vi "PCO_LensControlParameters.vi"() -> (0 "PCO_LensControlParameters":T2 {"dwStatusFlags" format="%x"}, 1 "PCO_LensControlParameters_Raw":T1, 2 "Length":u16, 3 "Raw_Length":u16)   [LabVIEW 2020, in "SDK.lvlib" / "Structures.lvlib"]
doc: "Use this template to build a VI to use as a subVI."
uses:
  Structures.lvlib
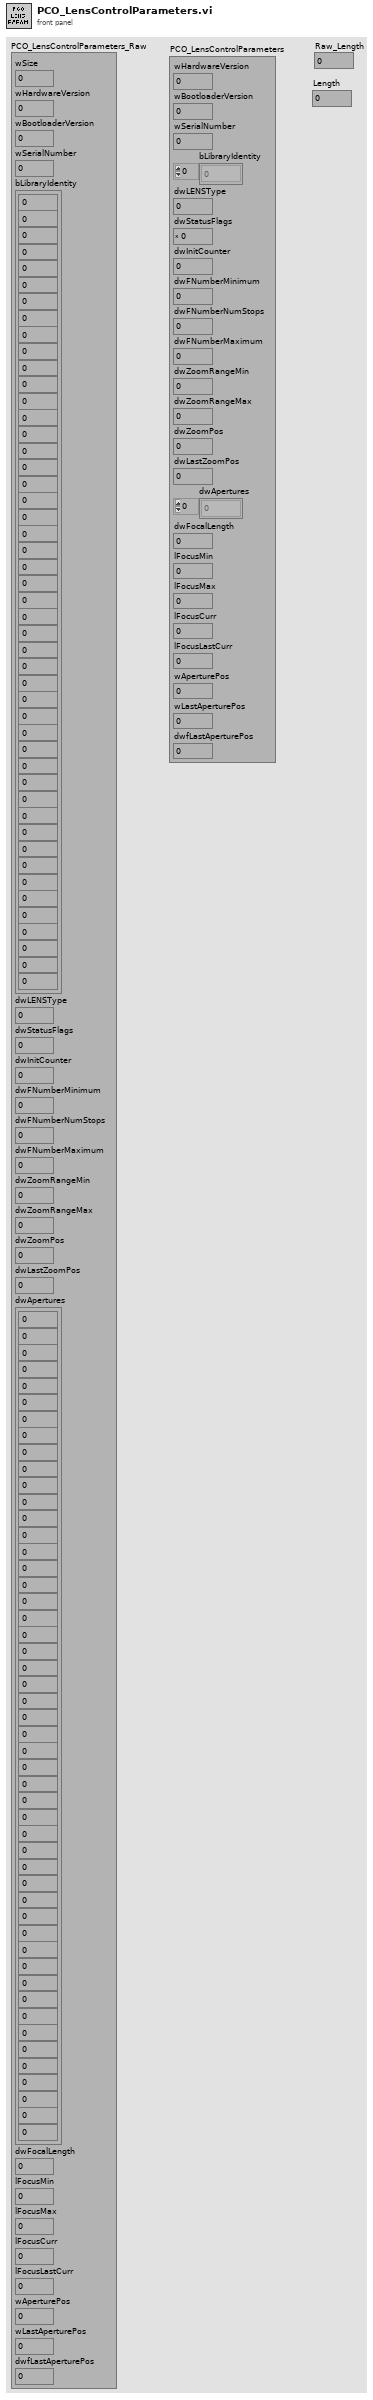
[diagram p1: front panel]
types:
  T1 = cluster{"wSize":u16, "wHardwareVersion":u16, "wBootloaderVersion":u16, "wSerialNumber":u16, "bLibraryIdentity":cluster{u8, u8, u8, u8, u8, u8, u8, u8, u8, u8, u8, u8, u8, u8, u8, u8, u8, u8, u8, u8, u8, u8, u8, u8, u8, u8, u8, u8, u8, u8, u8, u8, u8, u8, u8, u8, u8, u8, u8, u8, u8, u8, u8, u8, u8, u8, u8, u8}, "dwLENSType":u32, "dwStatusFlags":u32, "dwInitCounter":u32, "dwFNumberMinimum":u32, "dwFNumberNumStops":u32, "dwFNumberMaximum":u32, "dwZoomRangeMin":u32, "dwZoomRangeMax":u32, "dwZoomPos":u32, "dwLastZoomPos":u32, "dwApertures":cluster{u32, u32, u32, u32, u32, u32, u32, u32, u32, u32, u32, u32, u32, u32, u32, u32, u32, u32, u32, u32, u32, u32, u32, u32, u32, u32, u32, u32, u32, u32, u32, u32, u32, u32, u32, u32, u32, u32, u32, u32, u32, u32, u32, u32, u32, u32, u32, u32, u32, u32}, "dwFocalLength":u32, "lFocusMin":i32, "lFocusMax":i32, "lFocusCurr":i32, "lFocusLastCurr":i32, "wAperturePos":u16, "wLastAperturePos":u16, "dwfLastAperturePos":u32}
  T2 = cluster{"wHardwareVersion":u16, "wBootloaderVersion":u16, "wSerialNumber":u16, "bLibraryIdentity":u8[], "dwLENSType":u32, "dwStatusFlags":u32, "dwInitCounter":u32, "dwFNumberMinimum":u32, "dwFNumberNumStops":u32, "dwFNumberMaximum":u32, "dwZoomRangeMin":u32, "dwZoomRangeMax":u32, "dwZoomPos":u32, "dwLastZoomPos":u32, "dwApertures":u32[], "dwFocalLength":u32, "lFocusMin":i32, "lFocusMax":i32, "lFocusCurr":i32, "lFocusLastCurr":i32, "wAperturePos":u16, "wLastAperturePos":u16, "dwfLastAperturePos":u32}
  T3 = cluster{u32, u32, u32, u32, u32, u32, u32, u32, u32, u32, u32, u32, u32, u32, u32, u32, u32, u32, u32, u32, u32, u32, u32, u32, u32, u32, u32, u32, u32, u32, u32, u32, u32, u32, u32, u32, u32, u32, u32, u32, u32, u32, u32, u32, u32, u32, u32, u32, u32, u32}
  T4 = cluster{u8, u8, u8, u8, u8, u8, u8, u8, u8, u8, u8, u8, u8, u8, u8, u8, u8, u8, u8, u8, u8, u8, u8, u8, u8, u8, u8, u8, u8, u8, u8, u8, u8, u8, u8, u8, u8, u8, u8, u8, u8, u8, u8, u8, u8, u8, u8, u8}
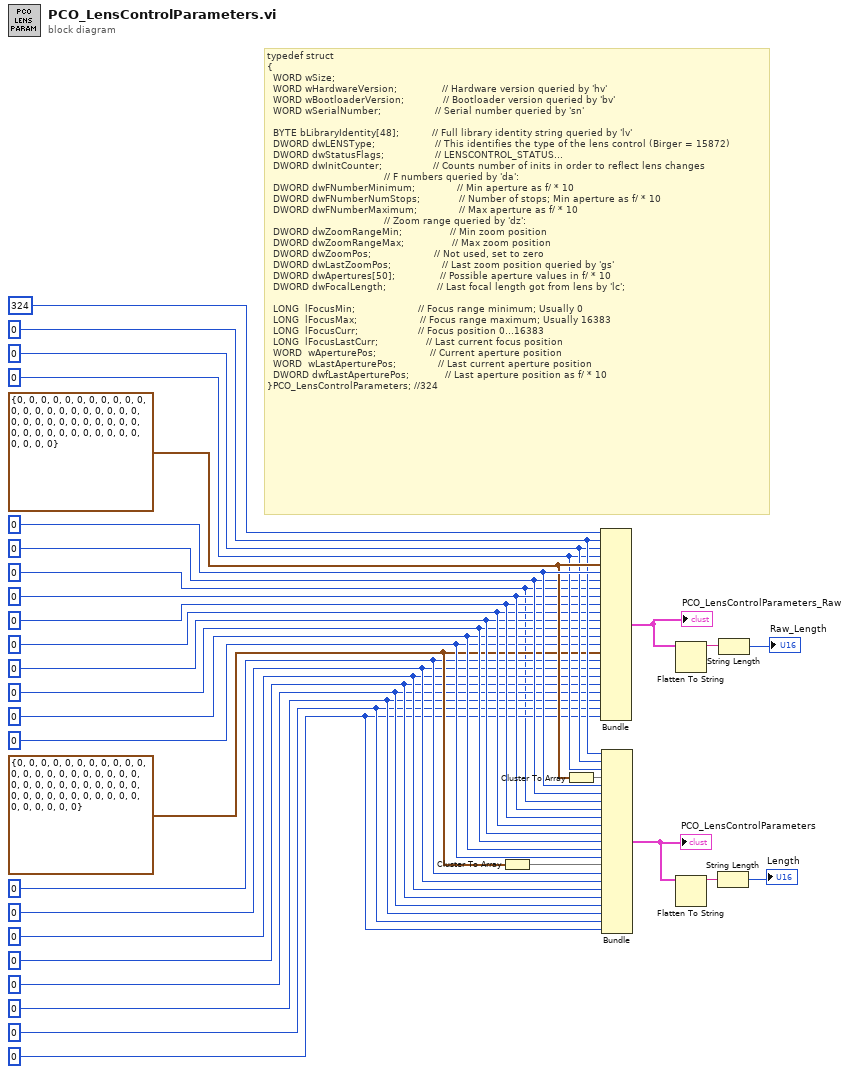
[diagram p0: block diagram]
diagram:
  w2 = u32 0 ("dwfLastAperturePos")
  w3 = u16 0 ("wLastAperturePos")
  w4 = u16 0 ("wAperturePos")
  w5 = 0 ("lFocusLastCurr")
  w6 = 0 ("lFocusCurr")
  w7 = 0 ("lFocusMax")
  w8 = 0 ("lFocusMin")
  w9 = u32 0 ("dwFocalLength")
  w11 = T3 {0, 0, 0, 0, 0, 0, 0, 0, 0, 0, 0, 0, 0, 0, 0, 0, 0, 0, 0, 0, 0, 0, 0, 0, 0, 0, 0, 0, 0, 0, 0, 0, 0, 0, 0, 0, 0, 0, 0, 0, 0, 0, 0, 0, 0, 0, 0, 0, 0, 0} ("dwApertures")
  w12 = u32 0 ("dwLastZoomPos")
  w13 = u32 0 ("dwZoomPos")
  w24 = T4 {0, 0, 0, 0, 0, 0, 0, 0, 0, 0, 0, 0, 0, 0, 0, 0, 0, 0, 0, 0, 0, 0, 0, 0, 0, 0, 0, 0, 0, 0, 0, 0, 0, 0, 0, 0, 0, 0, 0, 0, 0, 0, 0, 0, 0, 0, 0, 0} ("bLibraryIdentity")
  w14 = u32 0 ("dwZoomRangeMax")
  w15 = u32 0 ("dwZoomRangeMin")
  w16 = u32 0 ("dwFNumberMaximum")
  w17 = u32 0 ("dwFNumberNumStops")
  w18 = u32 0 ("dwFNumberMinimum")
  w1 = u32 0 ("dwInitCounter")
  w19 = u32 0 ("dwStatusFlags")
  w26 = u32 0 ("dwLENSType")
  w20 = u16 0 ("wSerialNumber")
  w21 = u16 0 ("wBootloaderVersion")
  w22 = u16 0 ("wHardwareVersion")
  # "typedef struct\n{\n  WORD wSize;\n  WORD wHardwareVersion;               // Hardware version queried by 'hv'\n  WORD wBootloaderVersion;             // Bootloader version queried by 'bv'\n  WORD wSerialNumber;                  // Serial number queried by 'sn'\n\n  BYTE bLibraryIdentity[48];           // Full library identity string queried by 'lv'\n  DWORD dwLENSType;                    // This identifies the type of the lens control (Birger = 15872)\n  DWORD dwStatusFlags;                 // LENSCONTROL_STATUS...\n  DWORD dwInitCounter;                 // Counts number of inits in order to reflect lens changes\n                                       // F numbers queried by 'da':\n  DWORD dwFNumberMinimum;              // Min aperture as f/ * 10\n  DWORD dwFNumberNumStops;             // Number of stops; Min aperture as f/ * 10\n  DWORD dwFNumberMaximum;              // Max aperture as f/ * 10\n                                       // Zoom range queried by 'dz':\n  DWORD dwZoomRangeMin;                // Min zoom position\n  DWORD dwZoomRangeMax;                // Max zoom position\n  DWORD dwZoomPos;                     // Not used, set to zero\n  DWORD dwLastZoomPos;                 // Last zoom position queried by 'gs'\n  DWORD dwApertures[50];               // Possible aperture values in f/ * 10\n  DWORD dwFocalLength;                 // Last focal length got from lens by 'lc';\n\n  LONG  lFocusMin;                     // Focus range minimum; Usually 0\n  LONG  lFocusMax;                     // Focus range maximum; Usually 16383\n  LONG  lFocusCurr;                    // Focus position 0...16383\n  LONG  lFocusLastCurr;                // Last current focus position\n  WORD  wAperturePos;                  // Current aperture position\n  WORD  wLastAperturePos;              // Last current aperture position\n  DWORD dwfLastAperturePos;            // Last aperture position as f/ * 10\n}PCO_LensControlParameters; //324"
  n1 = Cluster To Array(cluster=w11) -> (array=w10:u32[])
  n2 = Cluster To Array(cluster=w24) -> (array=w23:u8[])
  n3 = Bundle("wSize"=u16 324, "wHardwareVersion"=w22, "wBootloaderVersion"=w21, "wSerialNumber"=w20, "bLibraryIdentity"=w24, "dwLENSType"=w26, "dwStatusFlags"=w19, "dwInitCounter"=w1, "dwFNumberMinimum"=w18, "dwFNumberNumStops"=w17, "dwFNumberMaximum"=w16, "dwZoomRangeMin"=w15, "dwZoomRangeMax"=w14, "dwZoomPos"=w13, "dwLastZoomPos"=w12, "dwApertures"=w11, "dwFocalLength"=w9, "lFocusMin"=w8, "lFocusMax"=w7, "lFocusCurr"=w6, "lFocusLastCurr"=w5, "wAperturePos"=w4, "wLastAperturePos"=w3, "dwfLastAperturePos"=w2) -> (w27:T1)  [unwired: 1 in]
  "PCO_LensControlParameters_Raw" <- w27
  n4 = Bundle("wHardwareVersion"=w22, "wBootloaderVersion"=w21, "wSerialNumber"=w20, "bLibraryIdentity"=w23, "dwLENSType"=w26, "dwStatusFlags"=w19, "dwInitCounter"=w1, "dwFNumberMinimum"=w18, "dwFNumberNumStops"=w17, "dwFNumberMaximum"=w16, "dwZoomRangeMin"=w15, "dwZoomRangeMax"=w14, "dwZoomPos"=w13, "dwLastZoomPos"=w12, "dwApertures"=w10, "dwFocalLength"=w9, "lFocusMin"=w8, "lFocusMax"=w7, "lFocusCurr"=w6, "lFocusLastCurr"=w5, "wAperturePos"=w4, "wLastAperturePos"=w3, "dwfLastAperturePos"=w2) -> (w25:T2)  [unwired: 1 in]
  "PCO_LensControlParameters" <- w25
  n5 = Flatten To String(anything=w27) -> (data string=w31:string)  [unwired: 3 in, 2 out]
  n6 = Flatten To String(anything=w25) -> (data string=w32:string)  [unwired: 3 in, 2 out]
  n7 = String Length(string=w32) -> (length=→"Length":i32)
  n8 = String Length(string=w31) -> (length=→"Raw_Length":i32)
